vi "Read Lines Until Code Rcvd.vi"(8 "error in (no error)":errorcluster, 11 "FTP in":refnum<class "FTP.lvclass">) -> (0 "error out":errorcluster, 2 "String":string, 3 "FTP out":refnum<class "FTP.lvclass">)   [LabVIEW 2014, in "FTP.lvlib" / "FTP.lvclass"]
uses:
  FTP.lvclass
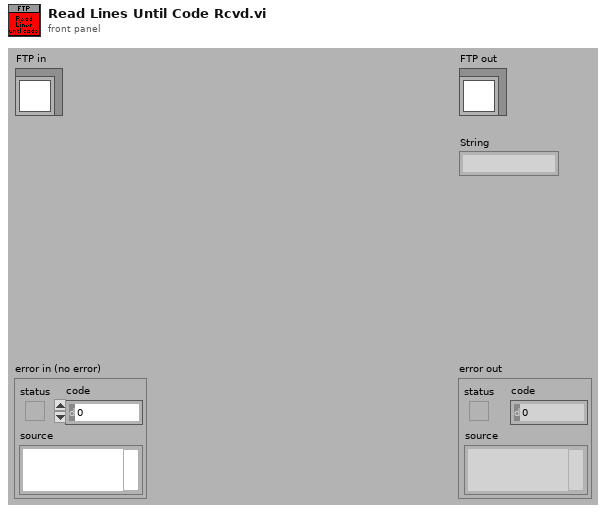
[diagram p1: front panel]
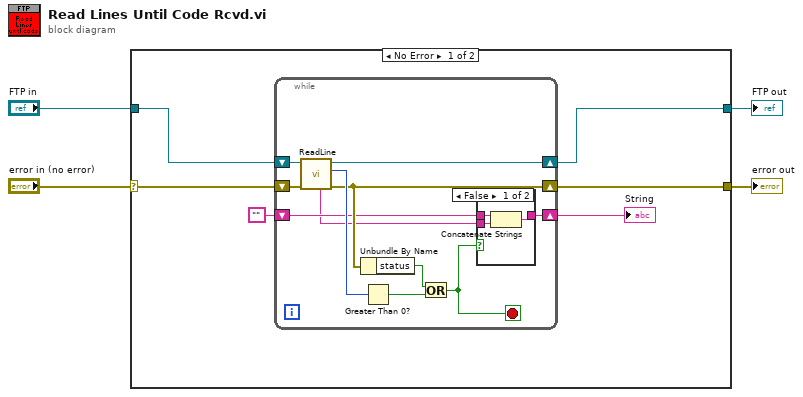
[diagram p0: block diagram]
diagram:
  n1 = case shown="No Error" "error in (no error)" {
    selector: "error in (no error)" -> [w9 w27]
    tunnel: [w6 w27] -> w3
    tunnel: [w7 w26] -> w1
    tunnel: "FTP in" -> [w8 w26]
    frame No Error {
      n2 = while {
        shift-right: [w19] -> w7
        shift-left: w8 -> [w21]
        shift-right: [w16] -> w6
        shift-left: w9 -> [w20]
        shift-right: [w13] -> w5
        shift-left: "" -> [w14]
        stop <- w12 stop-if-true
        n3 = call "ReadLine.vi"("error in (no error)"=w20, "FTP in"=w21) -> ("error out"=w16:errorcluster, "code"=w18:i32, "FTP out"=w19:refnum<class "FTP.lvclass">, "Full Line"=w11:string)  [unwired: 5 in, 1 out]
        n4 = Unbundle By Name(w16) -> ("status"=w15:bool)
        n5 = Greater Than 0?(x=w18) -> (x > 0?=w17:bool)
        n6 = Or(x=w15, y=w17) -> (x .or. y?=w12:bool)
        n7 = case shown="False" w12 {
          tunnel: w14 -> [w24 w25]
          tunnel: w11 -> [w23 _]
          tunnel: [w22 w25] -> w13
          frame False {
            n8 = Concatenate Strings(w24, w23) -> (w22:string)
          }
          frame True {
          }
        }
      }
      "String" <- w5
    }
    frame Error {
    }
  }
  "error out" <- w3
  "FTP out" <- w1
